vi "RollValidate.vi"() -> ()   [LabVIEW 2016]
uses:
  <vilib>/Platform/TimedLoop/XDataNode/timing_clust.ctl
  <vilib>/Platform/TimedLoop/XDataNode/nitl_modes.ctl
  <vilib>/Platform/TimedLoop/XDataNode/wakeup.ctl
  <vilib>/myRIO/Instrument Drivers/Onboard IO/PWM/typedefs/PWM Reference.ctl
  <vilib>/myRIO/Common/Instrument Driver Framework/Utilities/typedefs/myRIO Generic Hardware Reference.ctl
  <vilib>/myRIO/Common/Instrument Driver Framework/Utilities/typedefs/Hardware Version Enum.ctl
  <vilib>/myRIO/Common/Instrument Driver Framework/Utilities/typedefs/myRIO v1.0 Reference.ctl
  <vilib>/myRIO/Common/Instrument Driver Framework/Utilities/typedefs/Generic FPGA Reference.ctl
  <vilib>/myRIO/Common/Instrument Driver Framework/myRIO v1.0/PWM/typedefs/PWM Channels Enum.ctl
  <vilib>/myRIO/Instrument Drivers/Onboard IO/PWM/typedefs/PWM Configuration.ctl
  <vilib>/userdefined/High Color/nirio_resource_hc.ctl
  <vilib>/myRIO/Instrument Drivers/Onboard IO/AI/typedefs/AI Reference.ctl
  <vilib>/myRIO/Common/Instrument Driver Framework/myRIO v1.0/AI/typedefs/AI Channels List.ctl
  <vilib>/myRIO/Common/Instrument Driver Framework/myRIO v1.0/AI/typedefs/AI Channels Enum.ctl
  <vilib>/myRIO/Common/Instrument Driver Framework/Utilities/typedefs/Analog Scaling Constants List.ctl
  <vilib>/myRIO/Common/Instrument Driver Framework/Utilities/typedefs/Analog Scaling Constants.ctl
  <vilib>/myRIO/Common/Instrument Driver Framework/Utilities/vis/Is FPGA Ref Available.vi
  <vilib>/myRIO/Common/Instrument Driver Framework/roboRIO v1.0/AI/vis/roboRIO v1.0 Open AI.vi
  <vilib>/myRIO/Instrument Drivers/Onboard IO/AI/vis/Read.vi
  <vilib>/myRIO/Common/Instrument Driver Framework/roboRIO v1.0/PWM/vis/roboRIO v1.0 Open PWM.vi
  <vilib>/myRIO/Instrument Drivers/Onboard IO/PWM/vis/Set Duty Cycle and Frequency.vi
  <vilib>/myRIO/Common/Instrument Driver Framework/Utilities/vis/Validate Channels.vi
  <vilib>/myRIO/Common/Instrument Driver Framework/roboRIO v1.0/AI/vis/roboRIO v1.0 Reserve AI.vi
  <vilib>/myRIO/Common/Instrument Driver Framework/roboRIO v1.0/PWM/vis/roboRIO v1.0 Reserve PWM.vi
  <vilib>/myRIO/Common/Instrument Driver Framework/roboRIO v1.0/Resource Manager/vis/roboRIO v1.0 Reserve Channel List.vi
  <vilib>/myRIO/Common/Instrument Driver Framework/roboRIO v1.0/AI/vis/roboRIO v1.0 Build MUX Configuration AI.vi
  <vilib>/myRIO/Common/Instrument Driver Framework/roboRIO v1.0/PWM/vis/roboRIO v1.0 Build MUX Configuration PWM.vi
  <vilib>/myRIO/Common/Instrument Driver Framework/roboRIO v1.0/Resource Manager/vis/roboRIO v1.0 Reserve Channel.vi
  <vilib>/myRIO/Common/Instrument Driver Framework/roboRIO v1.0/Resource Manager/vis/roboRIO v1.0 Unreserve Channel.vi
  <vilib>/myRIO/Common/Instrument Driver Framework/roboRIO v1.0/Resource Manager/vis/roboRIO v1.0 Create Configuration List.vi
  <vilib>/myRIO/Common/Instrument Driver Framework/roboRIO v1.0/Resource Manager/vis/roboRIO v1.0 Build Mutex Name.vi
  <vilib>/Utility/VariantDataType/GetNumericInfo.vi
  <vilib>/Utility/error.llb/Error Cluster From Error Code.vi
  <vilib>/myRIO/Common/Instrument Driver Framework/roboRIO v1.0/roboRIO v1.0 Open.vi
  <vilib>/myRIO/Common/Instrument Driver Framework/Utilities/vis/IO Manager.vi
  <vilib>/myRIO/Common/Instrument Driver Framework/Utilities/vis/Configuration Manager.vi
  <vilib>/myRIO/Common/Instrument Driver Framework/roboRIO v1.0/Resource Manager/vis/roboRIO v1.0 Configure IO.vi
  <vilib>/myRIO/Common/Instrument Driver Framework/myRIO v1.0/myRIO v1.0 Close.vi
  <vilib>/myRIO/Common/Instrument Driver Framework/roboRIO v1.0/PWM/vis/roboRIO v1.0 Write PWM.vi
  <vilib>/myRIO/Common/Instrument Driver Framework/roboRIO v1.0/AI/vis/roboRIO v1.0 Get Scaling Constants AI.vi
  <vilib>/myRIO/Common/Instrument Driver Framework/roboRIO v1.0/AI/vis/roboRIO v1.0 Read AI.vi
  <vilib>/Platform/TimedLoop/XDataNode/XDataNode.xnode
  <vilib>/myRIO/Express VI/Onboard IO/PWM/PWM Express VI.xnode
  <vilib>/myRIO/Instrument Drivers/Onboard IO/PWM/vis/myRIO PWM Open.xnode
  <vilib>/myRIO/Express VI/Onboard IO/AI/AI Express VI.xnode
  <vilib>/myRIO/Instrument Drivers/Onboard IO/AI/vis/myRIO AI Open.xnode
  <vilib>/Platform/TimedLoop/XDataNode/XDNodeRunTimeDep.lvlib
  <vilib>/myRIO/Instrument Drivers/Onboard IO/PWM/PWM.lvlib
  <vilib>/myRIO/Instrument Drivers/Onboard IO/AI/AI.lvlib
panel:
  in  "SteeringAngle":dbl
  in  "v":dbl
  in  "Goal Degree":dbl=31.0 min=-90.0 max=90.0 step=5.0
  out "Laser On Diod":bool
  out "Photo diod value":dbl
  out "ms":dbl
  out "Duty Cycle":dbl
  in  "Degree":dbl=31.0 min=-90.0 max=90.0 step=5.0
  out "Bias":T1
  in  "stop":bool
  out "error out":errorcluster
  in  "Start":bool
  out "Roll":dbl
  out "IMU loop finished late":bool
  out "Roll & Pitch":dbl(graph)
  out "IMU loop lates":i32
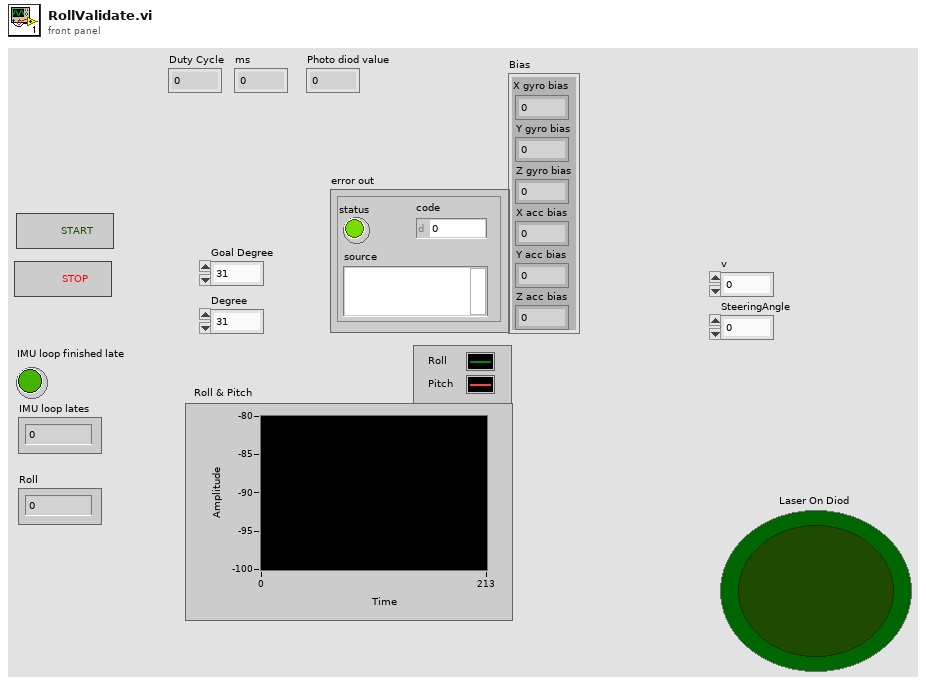
[diagram p1: front panel]
types:
  T1 = cluster{"X gyro bias":dbl, "Y gyro bias":dbl, "Z gyro bias":dbl, "X acc bias":dbl, "Y acc bias":dbl, "Z acc bias":dbl}
  T2 = enum16{"open", "open or create", "create or replace", "create", "open (read-only)"}
  T3 = cluster{"FilteredGyroX":dbl, "FilteredGyroY":dbl}
  T4 = typedef "AI.lvlib/AI Reference.ctl" = cluster{"myRIO Reference":T5, "AI Channels List":T9, "AI Scaling Constants List":T11}
  T5 = typedef "myRIO Generic Hardware Reference.ctl" = cluster{"myRIO Model":T6, "myRIO Hardware Reference":T7}
  T6 = typedef "Hardware Version Enum.ctl" = enum16{"Unknown", "myRIO-1900", "myRIO-1950", "roboRIO", "NI ELVIS RIO CM"}
  T7 = typedef "myRIO v1.0 Reference.ctl" = cluster{"Generic FPGA Reference":T8, "Allow multiple opens":bool}
  T8 = typedef "Generic FPGA Reference.ctl" = refnum<k20>
  T9 = typedef "AI Channels List.ctl" = T10[]
  T10 = typedef "AI Channels Enum.ctl" = enum16{"Not Connected", "AudioIn/Left", "AudioIn/Right", "C/AI0", "C/AI1", "A/AI0", "A/AI1", "A/AI2", "A/AI3", "B/AI0", "B/AI1", "B/AI2", "B/AI3", "AI/AI0", "AI/AI1", "AI/AI2", "AI/AI3"}
  T11 = typedef "Analog Scaling Constants List.ctl" = T12[]
  T12 = typedef "Analog Scaling Constants.ctl" = cluster{"LSB Weight (Volts)":dbl, "Offset (Volts)":dbl, "Signed?":bool}
  T13 = typedef "nirio_resource_hc.ctl" = tag
  T14 = typedef "PWM.lvlib/PWM Reference.ctl" = cluster{"myRIO Reference":T5, "PWM Channels Enum":T15, "PWM Configuration":T16}
  T15 = typedef "PWM Channels Enum.ctl" = enum16{"Not Connected", "C/PWM0", "C/PWM1", "A/PWM0", "A/PWM1", "A/PWM2", "B/PWM0", "B/PWM1", "B/PWM2", "PWM/PWM0", "PWM/PWM1", "PWM/PWM2", "PWM/PWM3", "PWM/PWM4", "PWM/PWM5", "PWM/PWM6", "PWM/PWM7", "PWM/PWM8", "PWM/PWM9"}
  T16 = typedef "PWM.lvlib/PWM Configuration.ctl" = cluster{"Frequency":dbl, "Duty Cycle":dbl}
  T17 = typedef "XDNodeRunTimeDep.lvlib/timing_clust.ctl" = cluster{"Expected End [f-1]":u64, "Actual End [f-1]":u64, "Finished Late? [f-1]":bool, "Expected End [i-1]":u64, "Actual End [i-1]":u64, "Finished Late? [i-1]":bool, "Expected Start [i]":u64, "Actual Start [i]":u64, "Expected Start [f]":u64, "Actual Start [f]":u64, "Source Name":string, "Structure Name":string, "Period":i64, "Deadline":i64, "Offset":i64, "Start":i64, "Priority":i32, "Timeout":i32, "Mode":T18, "Wakeup Reason":T19, "Error":errorcluster, "Source Type":string, "Secondary Source Type":string, "Global End Time":u64, "Global Start Time":u64, "Frame Duration":u64, "Iteration Duration":u64, "Assigned CPU":i32, "I/O Scan Engine Mode":u32}
  T18 = typedef "XDNodeRunTimeDep.lvlib/nitl_modes.ctl" = enum32{"No Change", "Process missed periods, maintain original phase", "Discard missed periods, maintain original phase", "Process missed periods, ignore original phase", "Discard missed periods, ignore original phase"}
  T19 = typedef "XDNodeRunTimeDep.lvlib/wakeup.ctl" = enum32{"Normal", "Aborted", "Asynchronous wakeup", "Timing source error", "Timed loop error", "Timeout"}
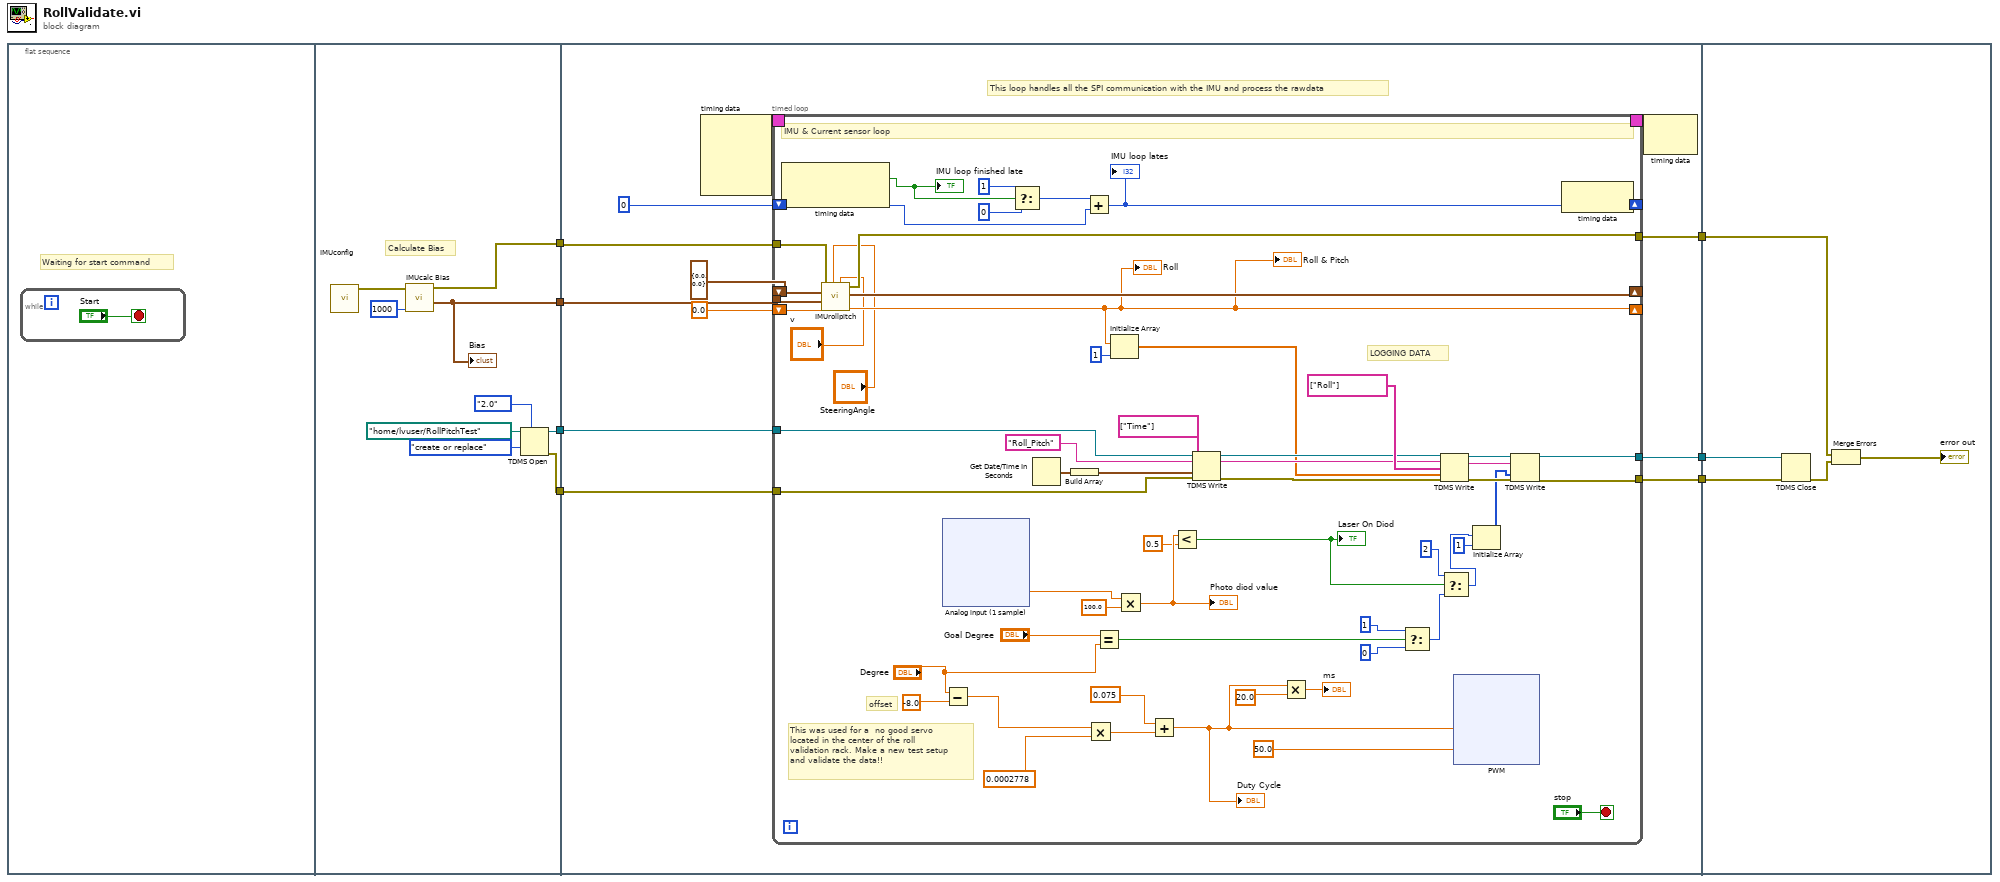
[diagram p0: block diagram]
diagram:
  n1 = flat-sequence {
    tunnel: [w17] -> w7
    tunnel: [w16] -> w6
    tunnel: [w14] -> w5
    tunnel: [w13] -> w4
    tunnel: w7 -> [w25]
    tunnel: w6 -> [w24]
    tunnel: w5 -> [w23]
    tunnel: w4 -> [w22]
    tunnel: [w21] -> w3
    tunnel: [w20] -> w2
    tunnel: [w19] -> w1
    tunnel: w3 -> [w167]
    tunnel: w2 -> [w166]
    tunnel: w1 -> [w165]
    frame #0 {
      # "Waiting for start command"
      n2 = while {
        stop <- "Start" stop-if-true
      }
    }
    frame #1 {
      # "Calculate Bias"
      n3 = call "IMUconfig.vi"() -> ("error out"=w9:errorcluster)  [unwired: 11 in]
      n4 = call "IMUcalc Bias.vi"("Number of loops"=1000, "error in (no error)"=w9) -> ("Bias"=w17:T1, "error out"=w16:errorcluster)  [unwired: 7 in]
      "Bias" <- w17
      n5 = TDMS Open(7:enum16{"1.0", "2.0"}."2.0" ("file format version (2.0)"), 10:T2."create or replace" ("operation (0:open)"), 11:path "/home/lvuser/RollPitchTest" ("file path")) -> (0:w13:errorcluster, 3:w14:refnum<k34>)  [unwired: 4 in]
    }
    frame #2 {
      # "This loop handles all the SPI communication with the IMU and process the rawdata"
      n6 = node-c288() -> (w29:T17)  [unwired: 4 in]
      n7 = timed-loop {
        timing: w29 -> [_]
        timing-out: [_] -> w28
        tunnel: w25 -> [w37]
        tunnel: w24 -> [w86]
        shift-right: [w32] -> _
        shift-left: 0.0 ("xAngle in") -> [w36]
        tunnel: [w79] -> w19
        shift-right: [w81] -> _
        shift-left: 0 ("t") -> [w80]
        tunnel: w23 -> [w72]
        tunnel: w22 -> [w71]
        tunnel: [w43] -> w21
        tunnel: [w46] -> w20
        shift-right: [w35] -> _
        shift-left: T3 {"FilteredGyroX"=0.0, "FilteredGyroY"=0.0} ("FilteredGyro") -> [w33]
        stop <- "stop" stop-if-true
        # "This was used for a  no good servo \nlocated in the center of the roll\nvalidation rack. Make a new test setup\nand validate the data!!"
        # "offset"
        # "LOGGING DATA"
        # "IMU & Current sensor loop"
        n8 = node-c288() -> (w85:bool)  [unwired: 1 in, 1 out]
        "IMU loop finished late" <- w85
        n9 = call "IMUrollpitch.vi"("v(m/s)"="v", "SteeringAngle(rad/s)"="SteeringAngle", "PrevRoll(deg)"=w36, "Bias"=w37, "PrevFilteredGyro(deg)"=w33, "error in (no error)"=w86) -> ("Roll(deg)"=w32:dbl, "FilteredGyro(deg)"=w35:T3, "error out"=w79:errorcluster)  [unwired: 3 in]
        "Roll" <- w32
        "Roll & Pitch" <- w32
        n10 = xnode "Analog input (1 sample)"() -> ("B/AI3 (Pin 9)"=w57:dbl)  [unwired: 1 in, 1 out]
        n11 = Subtract(x="Degree", y=-8.0) -> (x-y=w59:dbl)
        n12 = Select(t=1, s=w85, f=0 ("t")) -> (s? t:f=w82:i32)
        n13 = Get Date/Time In Seconds() -> (seconds since 1Jan1904=w78:timestamp)
        n14 = Build Array(w78) -> (w77:timestamp[])
        n15 = Add(x=w82, y=w80) -> (x+y=w81:i32)
        "IMU loop lates" <- w81
        n16 = Multiply(x=w59, y=0.0002778) -> (x*y=w69:dbl)
        n17 = Equal?(x="Goal Degree", y="Degree") -> (x = y?=w52:bool)
        n18 = Initialize Array(w32, 1 ("dimension size")) -> (w34:dbl[])
        n19 = Multiply(x=w57, y=100.0) -> (x*y=w56:dbl)
        "Photo diod value" <- w56
        n20 = Add(x=0.075, y=w69) -> (x+y=w63:dbl)
        "Duty Cycle" <- w63
        n21 = Less?(x=w56, y=0.5) -> (x < y?=w47:bool)
        "Laser On Diod" <- w47
        n22 = TDMS Write(0:w72, 5:"Roll_Pitch" ("group name in (Untitled)"), 7:string[] ["Time"] ("channel name(s) in (Untitled)"), 9:w77, 11:w71) -> (4:w65:refnum<k34>, 6:w67:string, 15:w66:errorcluster)  [unwired: 1 in, 1 out]
        n23 = Multiply(x=w63, y=20.0) -> (x*y=→"ms":dbl)
        n24 = Select(t=1, s=w52, f=0) -> (s? t:f=w49:i32)
        n25 = TDMS Write(0:w65, 5:w67, 7:string[] ["Roll"] ("channel name(s) in (Untitled)"), 9:w34, 11:w66) -> (4:w44:refnum<k34>, 6:w42:string, 15:w45:errorcluster)  [unwired: 1 in, 1 out]
        n26 = Select(t=2, s=w47, f=w49) -> (s? t:f=w39:i32)
        n27 = xnode "PWM"("Duty Cycle"=w63, "Frequency [Hz]"=50.0) -> ()  [unwired: 1 in, 1 out]
        n28 = Initialize Array(w39, 1 ("dimension size")) -> (w41:i32[])
        n29 = TDMS Write(0:w44, 5:w42, 9:w41, 11:w45) -> (4:w43:refnum<k34>, 15:w46:errorcluster)  [unwired: 2 in, 2 out]
        n30 = node-c288() -> ()  [unwired: 1 in, 1 out]
      }
      n31 = node-c288(w28) -> ()  [unwired: 1 out]
    }
    frame #3 {
      n32 = TDMS Close(8:w166, 11:w167) -> (0:w168:errorcluster)  [unwired: 1 out]
      n33 = Merge Errors(w165, w168) -> (→"error out":errorcluster)
    }
  }
